vi "Write BaseNode ID.vi"(8 "error in (no error)":errorcluster, 10 "BaseNode ID":u64, 11 "Scalar Bitpacking Testing in":refnum<class "FPGA Addon Scalar Bitpacking Unit Tests.lvclass">) -> (0 "error out":errorcluster, 3 "Scalar Bitpacking Testing out":refnum<class "FPGA Addon Scalar Bitpacking Unit Tests.lvclass">)   [LabVIEW 2018, in "FPGA Addon Scalar Bitpacking Unit Tests.lvclass"]
uses:
  FPGA Addon Scalar Bitpacking Unit Tests.lvclass
  FPGA Addon Scalar Bitpacking Unit Tests.lvclass/FPGA Addon Scalar Bitpacking Unit Tests.ctl
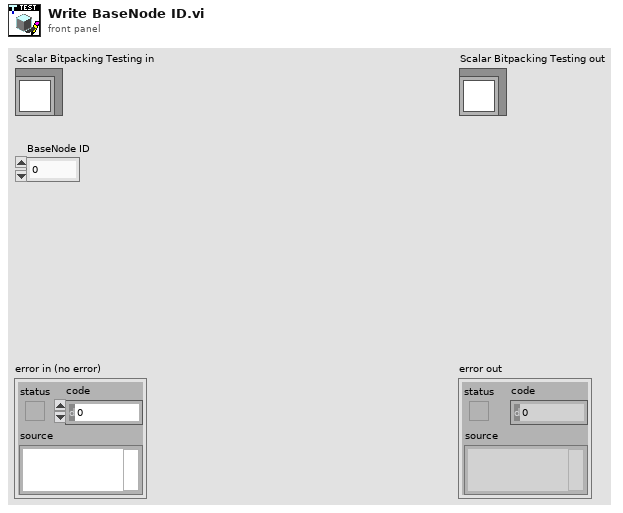
[diagram p1: front panel]
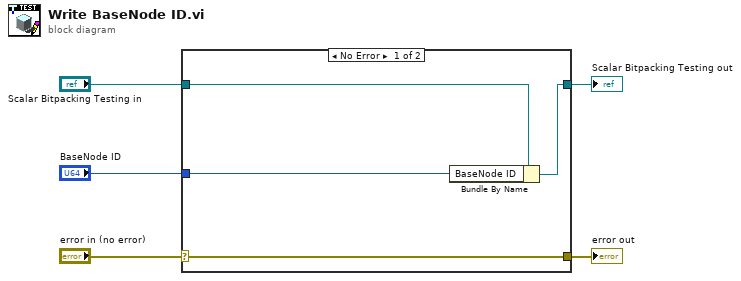
[diagram p0: block diagram]
diagram:
  n1 = case shown="No Error" "error in (no error)" {
    selector: "error in (no error)" -> [w9 w10]
    tunnel: [w9 w10] -> w4
    tunnel: [w7 w11] -> w2
    tunnel: "Scalar Bitpacking Testing in" -> [w8 w11]
    tunnel: "BaseNode ID" -> [w6 _]
    frame No Error {
      n2 = Bundle By Name(cluster=w8, "BaseNode ID"=w6) -> (w7:refnum<class "FPGA Addon Scalar Bitpacking Unit Tests.lvclass">)
    }
    frame Error {
    }
  }
  "error out" <- w4
  "Scalar Bitpacking Testing out" <- w2
